vi "add vectors.vi"(1 "vectors":cluster{"length":dbl, "angle":dbl}[](array[cluster])) -> (0 "vector":cluster{"length":dbl, "angle":dbl})   [LabVIEW 2009]
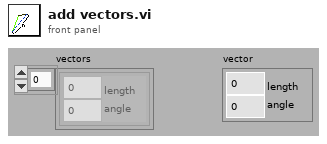
[diagram p1: front panel]
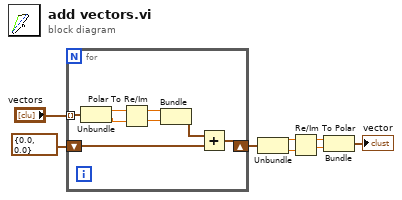
[diagram p0: block diagram]
diagram:
  n1 = for {
    tunnel: "vectors" -> [w16] mode=indexing
    shift-right: [w9] -> w6
    shift-left: cluster{dbl, dbl} {0.0, 0.0} ("output cluster") -> [w10]
    n2 = Unbundle(w16) -> ("length"=w13:dbl, "angle"=w12:dbl)
    n3 = Polar To Re/Im(2:w12, 3:w13) -> (0:w15:dbl, 1:w14:dbl)
    n4 = Bundle(w14, w15) -> (w11:cluster{dbl, dbl})  [unwired: 1 in]
    n5 = Add(x=w11, y=w10) -> (x+y=w9:cluster{dbl, dbl})
  }
  n6 = Unbundle(w6) -> (w5:dbl, w4:dbl)
  n7 = Re/Im To Polar(2:w4, 3:w5) -> (0:w2:dbl, 1:w3:dbl)
  n8 = Bundle(w3, w2) -> (→"vector":cluster{dbl, dbl})  [unwired: 1 in]
